vi "Move piezo 2.vi"(4 "Initial voltage":sgl=0.4 min=0.1 max=5 step=0.1 format="%.1f", 6 "dV":sgl=0.4 min=0.1 max=5 step=0.1 format="%.1f", 8 "error in (no error)":errorcluster, 9 "V Range":sgl=0.4 min=0.1 max=5 step=0.1 format="%.1f", 10 "Current voltage in":sgl=0.4 min=0.1 max=5 step=0.1 format="%.1f", 11 "VISA Refnum in":refnum<visa-resource-name>) -> (0 "error out":errorcluster, 2 "Stop?":bool, 3 "Current voltage out":sgl)   [LabVIEW 2020]
doc: "Send command to piezo driver to increment its voltage. Determines if the Range voltage value has been reached; if so, sent True to Stop?."
uses:
  <vilib>/Instr/_visa.llb/VISA Configure Serial Port (Instr).vi
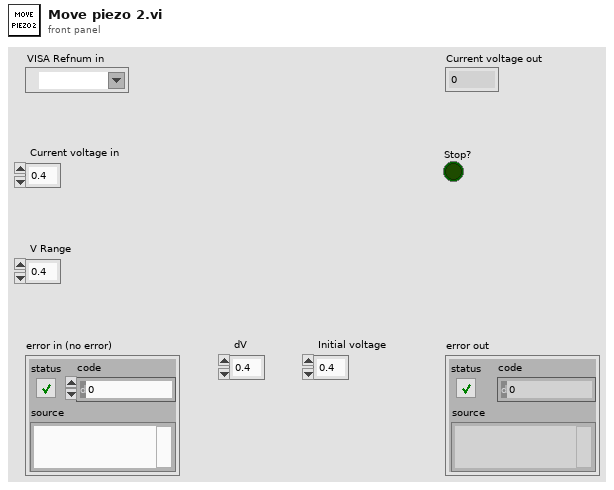
[diagram p1: front panel]
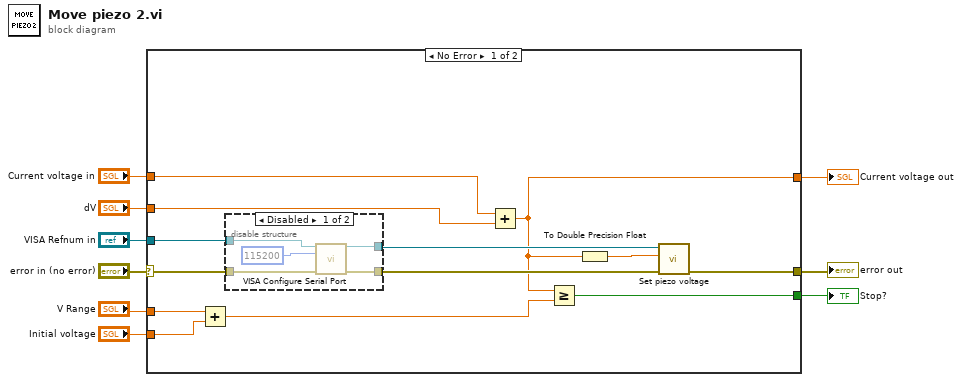
[diagram p0: block diagram]
diagram:
  n1 = case shown="No Error" "error in (no error)" {
    selector: "error in (no error)" -> [w21 w31]
    tunnel: "V Range" -> [w13 _]
    tunnel: "dV" -> [w14 _]
    tunnel: "VISA Refnum in" -> [w22 _]
    tunnel: [w18 w31] -> w6
    tunnel: [w20 _] -> w5
    tunnel: [w11 w30] -> w4
    tunnel: "Current voltage in" -> [w15 w30]
    tunnel: "Initial voltage" -> [w12 _]
    frame No Error {
      n2 = Add(x=w13, y=w12) -> (x+y=w10:sgl)
      n3 = disable-structure shown="Disabled" {
        disable-tunnel: w22 -> [w27 w28]
        disable-tunnel: w21 -> [w25 w29]
        disable-tunnel: [w24 w29] -> w19
        disable-tunnel: [w23 w28] -> w17
        frame Disabled {
          n4 = call-poly "VISA Configure Serial Port"("VISA resource name"=w27, "baud rate (9600)"=u32 115200, "error in (no error)"=w25) -> ("VISA resource name out"=w23:refnum<visa-resource-name>, "error out"=w24:errorcluster)  [unwired: 11 in]
        }
        frame Enabled {
        }
      }
      n5 = Add(x=w15, y=w14) -> (x+y=w11:sgl)
      n6 = Greater Or Equal?(x=w11, y=w10) -> (x >= y?=w20:bool)
      n7 = To Double Precision Float(number=w11) -> (double precision float=w16:dbl)
      n8 = call "Set piezo voltage.vi"("error in (no error)"=w19, "Voltage"=w16, "COM port in"=w17) -> ("error out"=w18:errorcluster)  [unwired: 7 in, 1 out]
    }
    frame Error {
    }
  }
  "error out" <- w6
  "Stop?" <- w5
  "Current voltage out" <- w4
